vi "Test_Image_Quality.vi"() -> ()   [LabVIEW 2017]
uses:
  <vilib>/userdefined/High Color/IMAQdx.ctl
  <vilib>/vision/driver/NI_Vision_Acquisition_Software.lvlib
  <vilib>/vision/NI_Vision_Development_Module.lvlib
panel:
  in  "Image Type":T1 items=["Grayscale (U8)", "Grayscale (I16)", "Grayscale (SGL)", "Complex (CSG)", "RGB (U32)", "HSL (U32)", "RGB (U64)", "Grayscale (U16)"]
  out "error out":errorcluster
  out "Within Range":bool
  out "Standard  Variation":sgl
  out "Mean Value":sgl
  out "Range":sgl
  out "Image":T2(plugin-control)
  in  "Session In":T3
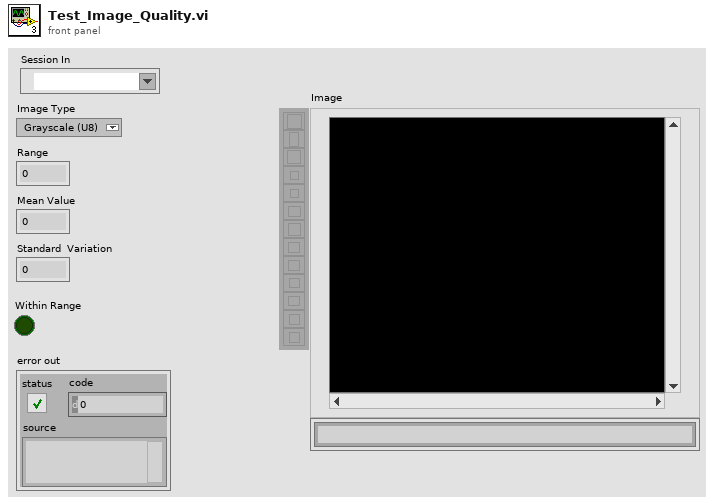
[diagram p1: front panel]
types:
  T1 = typedef "Image Type" = u32
  T2 = typedef "IMAQ Image.ctl" = refnum<image>
  T3 = typedef "IMAQdx.ctl" = refnum<k21>
  T4 = cluster{"histogram":u32[], "Minimal Value":sgl, "Maximal Value":sgl, "Starting Value":sgl, "Interval Width":sgl, "Mean Value":sgl, "Standard  Variation":sgl, "Area (pixels)":i32}
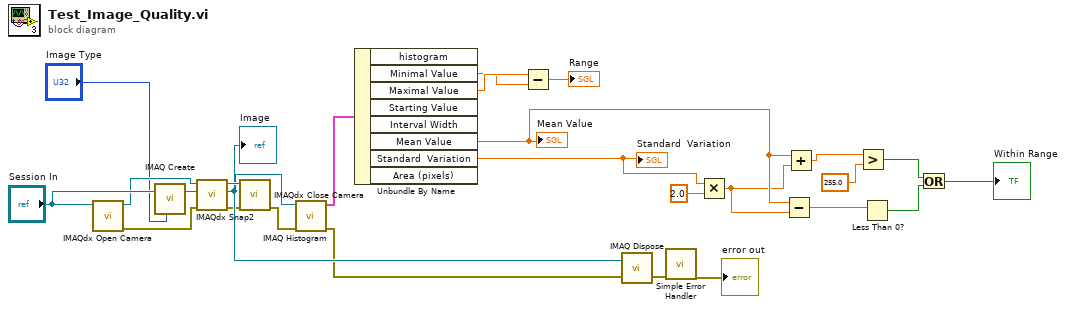
[diagram p0: block diagram]
diagram:
  n1 = call <vilib>:"IMAQdx Open Camera.vi"("Session In"="Session In") -> ("error out"=w22:errorcluster, "Session Out"=w25:T3)  [unwired: 9 in]
  n2 = call "IMAQ Create"("Image Name"="Session In", "Image Type"="Image Type") -> ("New Image"=w24:T2)  [unwired: 3 in, 1 out]
  n3 = call <vilib>:"IMAQdx Snap2.vi"("error in"=w22, "Image In"=w24, "Session In"=w25) -> ("error out"=w6:errorcluster, "Image Out"=w21:T2, "Session Out"=w23:T3)  [unwired: 6 in]
  "Image" <- w21
  n4 = call <vilib>:"IMAQdx Close Camera.vi"("error in"=w6, "Session In"=w23) -> ("error out"=w5:errorcluster)  [unwired: 9 in]
  n5 = call "IMAQ Histogram"("error in (no error)"=w5, "Image"=w21) -> ("error out"=w4:errorcluster, "Histogram Report"=w20:T4)  [unwired: 8 in]
  n6 = Unbundle By Name(w20) -> ("Minimal Value"=w18:sgl, "Maximal Value"=w19:sgl, "Mean Value"=w8:sgl, "Standard  Variation"=w15:sgl)  [unwired: 4 out]
  "Mean Value" <- w8
  "Standard  Variation" <- w15
  n7 = Subtract(x=w19, y=w18) -> (x-y=→"Range":sgl)
  n8 = call "IMAQ Dispose"("Image"=w21, "error in (no error)"=w4) -> ("error out"=w3:errorcluster)  [unwired: 4 in]
  n9 = call <vilib>:"Simple Error Handler.vi"("error in (no error)"=w3) -> ("error out"=→"error out":errorcluster)  [unwired: 4 in, 4 out]
  n10 = Multiply(x=w15, y=2.0) -> (x*y=w7:dbl)
  n11 = Subtract(x=w8, y=w7) -> (x-y=w9:dbl)
  n12 = Add(x=w8, y=w7) -> (x+y=w10:dbl)
  n13 = Greater?(x=w10, y=255.0) -> (0:w12:bool)
  n14 = Less Than 0?(x=w9) -> (x < 0?=w11:bool)
  n15 = Or(x=w12, y=w11) -> (x .or. y?=→"Within Range":bool)
